vi "TCP Read Length and Value (Array Dbl).vi"(8 "error in (no error)":errorcluster, 10 "timeout ms (1000)":i32=1000, 11 "TCP Network Connection in":refnum<k5>) -> (0 "error out":errorcluster, 2 "Output":dbl[](array[numeric]), 3 "TCP Network Connection out":refnum<k5>)   [LabVIEW 2019]
doc: "This software is licensed for use under the “MIT License\"\nCopyright (c) 2019 Scott Hannahs, sth@alum.mit.edu\n\nPermission is hereby granted, free of charge, to any person obtaining a copy of this software and associated documentation files (the \"Software\"), to deal in the Software without restriction, including without limitation the rights to use, copy, modify, merge, publish, distribute, sublicense, and/or sell copies of the Software, and to permit persons to whom the Software is furnished to do so, subject to the following conditions: The above copyright notice and this permission notice shall be included in all copies or substantial portions of the Software.\n\nTHE SOFTWARE IS PROVIDED \"AS IS\", WITHOUT WARRANTY OF ANY KIND, EXPRESS OR IMPLIED, INCLUDING BUT NOT LIMITED TO THE WARRANTIES OF MERCHANTABILITY, FITNESS FOR A PARTICULAR PURPOSE AND NONINFRINGEMENT. IN NO EVENT SHALL THE AUTHORS OR COPYRIGHT HOLDERS BE LIABLE FOR ANY CLAIM, DAMAGES OR OTHER LIABILITY, WHETHER IN AN ACTION OF CONTRACT, TORT OR OTHERWISE, ARISING FROM, OUT OF OR IN CONNECTION WITH THE SOFTWARE OR THE USE OR OTHER DEALINGS IN THE SOFTWARE."
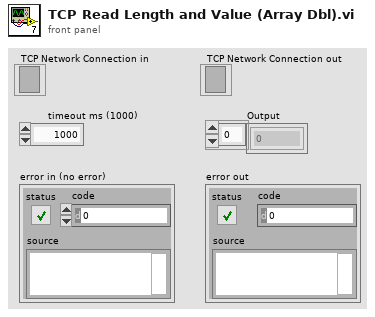
[diagram p1: front panel]
types:
  T1 = enum16{"Standard", "Buffered", "CRLF", "Immediate"}
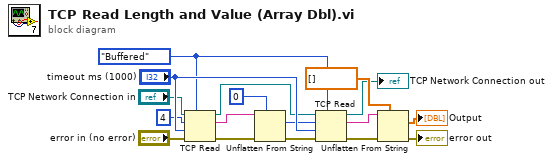
[diagram p0: block diagram]
diagram:
  w11 = T1."Buffered" ("mode (standard)")
  n1 = TCP Read(connection ID="TCP Network Connection in", bytes to read=u32 4, error in (no error)="error in (no error)", 7:w11, 9:"timeout ms (1000)") -> (connection ID out=w5:refnum<k5>, data out=w2:string, error out=w3:errorcluster)
  n2 = Unflatten From String(type=u32 0 ("bytes to read"), binary string=w2, error in (no error)=w3) -> (value=w6:u32, error out=w7:errorcluster)  [unwired: 2 in, 1 out]
  n3 = TCP Read(connection ID=w5, bytes to read=w6, error in (no error)=w7, 7:w11, 9:"timeout ms (1000)") -> (connection ID out=→"TCP Network Connection out":refnum<k5>, data out=w9:string, error out=w10:errorcluster)
  n4 = Unflatten From String(type=dbl[] [], binary string=w9, error in (no error)=w10) -> (value=→"Output":dbl[], error out=→"error out":errorcluster)  [unwired: 2 in, 1 out]
